vi "Read Cryogen Status.vi"() -> (1 "shutdown":bool, 2 "nitrogen":cluster{"fillN?":bool, "lowN?":bool} caption="Nitrogen", 3 "helium":T1 caption="Helium")   [LabVIEW 2009, in "Magnet.lvclass"]
uses:
  Magnet.lvclass
  Level Meter Setup.vi
  Level Meter.lvclass
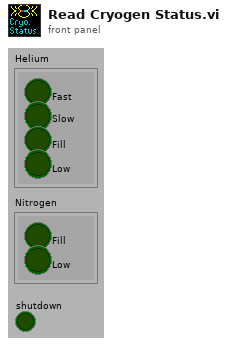
[diagram p1: front panel]
types:
  T1 = cluster{"fastHe?":bool, "slowHe?":bool, "fillHe?":bool, "lowHe?":bool}
  T2 = typedef "OxfordAddress.ctl" = cluster{"Com Port":i32, "ISOBUS Address":i32, "GPIB Address":i16, "Communication":enum16{"RS232", "ISOBUS", "GPIB", "Gateway"}}
  T3 = cluster{"Address":T2, "ILM Name":string, "Display Channel":i32[]}
  T4 = typedef "ILMRelayStatus.ctl" = cluster{"Shut down":bool, "Alarm sound":bool, "Alarm state":bool, "Silence prohib":bool, "Relay1 active":bool, "Relay 2 active":bool, "Relay 3 active":bool, "Relay 4 active":bool}
  T5 = typedef "ILMChannelStatus.ctl" = cluster{"Probe current":bool, "Probe fast":bool, "Probe slow":bool, "Auto-fill":enum16{"End fill", "Not filling", "Filling", "Start filling"}, "Fill":bool, "Low level":bool, "Alm requested":bool, "Pre-pulse I":bool}
  T6 = cluster{bool, bool, "Fill":bool, "Low level":bool}
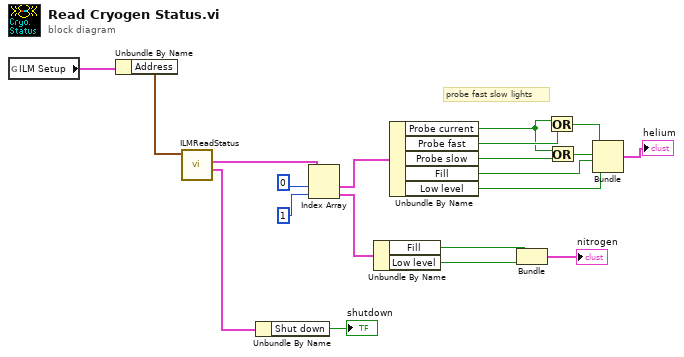
[diagram p0: block diagram]
diagram:
  # "probe fast slow lights"
  n1 = global read "Level Meter Setup.vi" "ILM Setup"() -> (w4:T3)
  n2 = Unbundle By Name(w4) -> ("Address"=w3:T2)
  n3 = call "ILMReadStatus.vi"("Instrument address"=w3) -> ("Relay"=w2:T4, "Channel"=w20:T5[])  [unwired: 5 out]
  n4 = Unbundle By Name(w2) -> ("Shut down"=→"shutdown":bool)
  n5 = Index Array(array=w20, index #1=0, index #2=1) -> (element #1=w17:T5, element #2=w16:T5)
  n6 = Unbundle By Name(w16) -> ("Fill"=w7:bool, "Low level"=w6:bool)
  n7 = Unbundle By Name(w17) -> ("Probe current"=w13:bool, "Probe fast"=w14:bool, "Probe slow"=w15:bool, "Fill"=w8:bool, "Low level"=w10:bool)
  n8 = Bundle("Fill"=w7, "Low level"=w6) -> (→"nitrogen":cluster{"Fill":bool, "Low level":bool})  [unwired: 1 out]
  n9 = Or(x=w13, y=w14) -> (x .or. y?=w11:bool)
  n10 = Or(x=w13, y=w15) -> (x .or. y?=w9:bool)
  n11 = Bundle(w11, w9, "Fill"=w8, "Low level"=w10) -> (→"helium":T6)  [unwired: 1 out]
